vi "get_shutter.vi"(8 "error in (no error)":errorcluster, 11 "LightSourceAN191011Chameleon in":refnum<class "LightSourceAN191011Chameleon.lvclass">) -> (0 "error out":errorcluster, 2 "shutter status":bool, 3 "LightSourceAN191011Chameleon out":refnum<class "LightSourceAN191011Chameleon.lvclass">)   [LabVIEW 2011, in "LightSourceAN191011Chameleon.lvclass"]
uses:
  LightSourceAN191011Chameleon.lvclass
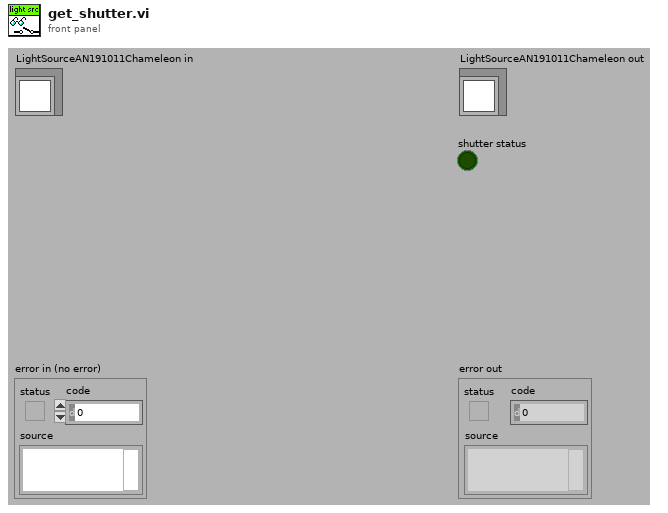
[diagram p1: front panel]
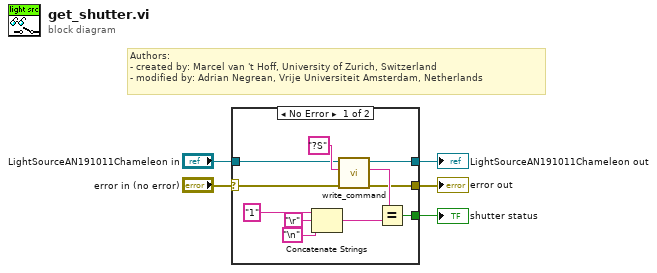
[diagram p0: block diagram]
diagram:
  # "Authors: \n- created by: Marcel van 't Hoff, University of Zurich, Switzerland\n- modified by: Adrian Negrean, Vrije Universiteit Amsterdam, Netherlands"
  n1 = case shown="No Error" "error in (no error)" {
    selector: "error in (no error)" -> [w8 w18]
    tunnel: [w7 w18] -> w4
    tunnel: [w9 w17] -> w2
    tunnel: "LightSourceAN191011Chameleon in" -> [w10 w17]
    tunnel: [w6 _] -> w1
    frame No Error {
      n2 = Concatenate Strings("1" ("y"), "\r", "\n") -> (w11:string)
      n3 = call-dynamic "write_command.vi"("error in (no error)"=w8, "string to write"="?S", "LightSourceAN191011Chameleon in"=w10) -> ("error out"=w7:errorcluster, "read string"=w15:string, "LightSourceAN191011Chameleon out"=w9:refnum<class "LightSourceAN191011Chameleon.lvclass">)  [unwired: 6 in]
      n4 = Equal?(x=w15, y=w11) -> (x = y?=w6:bool)
    }
    frame Error {
    }
  }
  "error out" <- w4
  "LightSourceAN191011Chameleon out" <- w2
  "shutter status" <- w1
